vi "Drive.vi"() -> (0 "Front Right":T1={"DeviceStatus"={"status"=FALSE, "code"=0, "source"=""}, "Type"=enum."PWM", "PWM"={"PWM Channel"=enum."PWM 1", "DeadBand"={"Name"="", "maxPositivePwm"=0, "minPositivePwm"=0, "centerPwm"=0, "maxNegativePwm"=0, "minNegativePwm"=0, "angularRange"=0}}, "CAN"={"Device Number"=0, "SetOutput VI Ref"=variant(enum8{"Percent VBus", "Current", "Speed", "Position", "Voltage"} enum."Percent VBus"), "GetOutput VI Ref"=variant(refnum<k1> refnum), "Enable VI Ref"=variant(dbl 12.0), "Disable VI Ref"=variant(enum8{"Percent VBus", "Speed", "Position", "Slave", "Unchanged / Invalid", "Voltage Compensation", "Current", "Motion Profile"} enum."Percent VBus"), "Data"=variant}, "Invert"=FALSE, "DIO PWM"={"PWM \"Enable\" Channel"=enum."Invalid", "DIOChannel"=enum."Invalid", "PWM Rate"=0.0}}, 1 "Front Left":T1={"DeviceStatus"={"status"=FALSE, "code"=0, "source"=""}, "Type"=enum."PWM", "PWM"={"PWM Channel"=enum."PWM 1", "DeadBand"={"Name"="", "maxPositivePwm"=0, "minPositivePwm"=0, "centerPwm"=0, "maxNegativePwm"=0, "minNegativePwm"=0, "angularRange"=0}}, "CAN"={"Device Number"=0, "SetOutput VI Ref"=variant(enum8{"Percent VBus", "Current", "Speed", "Position", "Voltage"} enum."Percent VBus"), "GetOutput VI Ref"=variant(refnum<k1> refnum), "Enable VI Ref"=variant(dbl 12.0), "Disable VI Ref"=variant(enum8{"Percent VBus", "Speed", "Position", "Slave", "Unchanged / Invalid", "Voltage Compensation", "Current", "Motion Profile"} enum."Percent VBus"), "Data"=variant}, "Invert"=FALSE, "DIO PWM"={"PWM \"Enable\" Channel"=enum."Invalid", "DIOChannel"=enum."Invalid", "PWM Rate"=0.0}}, 2 "Rear Right":T1={"DeviceStatus"={"status"=FALSE, "code"=0, "source"=""}, "Type"=enum."PWM", "PWM"={"PWM Channel"=enum."PWM 1", "DeadBand"={"Name"="", "maxPositivePwm"=0, "minPositivePwm"=0, "centerPwm"=0, "maxNegativePwm"=0, "minNegativePwm"=0, "angularRange"=0}}, "CAN"={"Device Number"=0, "SetOutput VI Ref"=variant(enum8{"Percent VBus", "Current", "Speed", "Position", "Voltage"} enum."Percent VBus"), "GetOutput VI Ref"=variant(refnum<k1> refnum), "Enable VI Ref"=variant(dbl 12.0), "Disable VI Ref"=variant(enum8{"Percent VBus", "Speed", "Position", "Slave", "Unchanged / Invalid", "Voltage Compensation", "Current", "Motion Profile"} enum."Percent VBus"), "Data"=variant}, "Invert"=FALSE, "DIO PWM"={"PWM \"Enable\" Channel"=enum."Invalid", "DIOChannel"=enum."Invalid", "PWM Rate"=0.0}}, 3 "Rear Left":T1={"DeviceStatus"={"status"=FALSE, "code"=0, "source"=""}, "Type"=enum."PWM", "PWM"={"PWM Channel"=enum."PWM 1", "DeadBand"={"Name"="", "maxPositivePwm"=0, "minPositivePwm"=0, "centerPwm"=0, "maxNegativePwm"=0, "minNegativePwm"=0, "angularRange"=0}}, "CAN"={"Device Number"=0, "SetOutput VI Ref"=variant(enum8{"Percent VBus", "Current", "Speed", "Position", "Voltage"} enum."Percent VBus"), "GetOutput VI Ref"=variant(refnum<k1> refnum), "Enable VI Ref"=variant(dbl 12.0), "Disable VI Ref"=variant(enum8{"Percent VBus", "Speed", "Position", "Slave", "Unchanged / Invalid", "Voltage Compensation", "Current", "Motion Profile"} enum."Percent VBus"), "Data"=variant}, "Invert"=FALSE, "DIO PWM"={"PWM \"Enable\" Channel"=enum."Invalid", "DIOChannel"=enum."Invalid", "PWM Rate"=0.0}})   [LabVIEW 2019]
uses:
  <vilib>/Rock Robotics/WPI/MotorControl/WPI_MotorControlDeviceRef.ctl
  <vilib>/Rock Robotics/WPI/MotorControl/WPI_MotorControlType.ctl
  <vilib>/Rock Robotics/SystemInterfaces/DIO/FPGA_DIOPWMChannel.ctl
  <vilib>/Rock Robotics/WPI/PWM/WPI_PWMDeadband.ctl
  <vilib>/Rock Robotics/SystemInterfaces/DIO/FPGA_DIOChannel.ctl
  <vilib>/Rock Robotics/WPI/ThirdParty/Phoenix-LabVIEW/Motor Controller/Controls/CTRE_Phoenix_MotorControl_ControlMode.ctl
  <vilib>/Rock Robotics/WPI/ThirdParty/Phoenix-LabVIEW/Motor Controller/Controls/CTRE_Phoenix_MotorControl_FeedbackDevice_TalonFX.ctl
  <vilib>/Rock Robotics/WPI/ThirdParty/Phoenix-LabVIEW/Motor Controller/Controls/CTRE_Phoenix_MotorControl_NeutralMode.ctl
  <vilib>/Rock Robotics/WPI/ThirdParty/Phoenix-LabVIEW/CANCoder/Controls/CTRE_Phoenix_CANcoder_SensorInitializationStrategy.ctl
  <vilib>/Rock Robotics/WPI/ThirdParty/Phoenix-LabVIEW/Motor Controller/Sensor/CTRE_Phoenix_MotorControl_SetIntegratedSensorPosition_TalonFX.vi
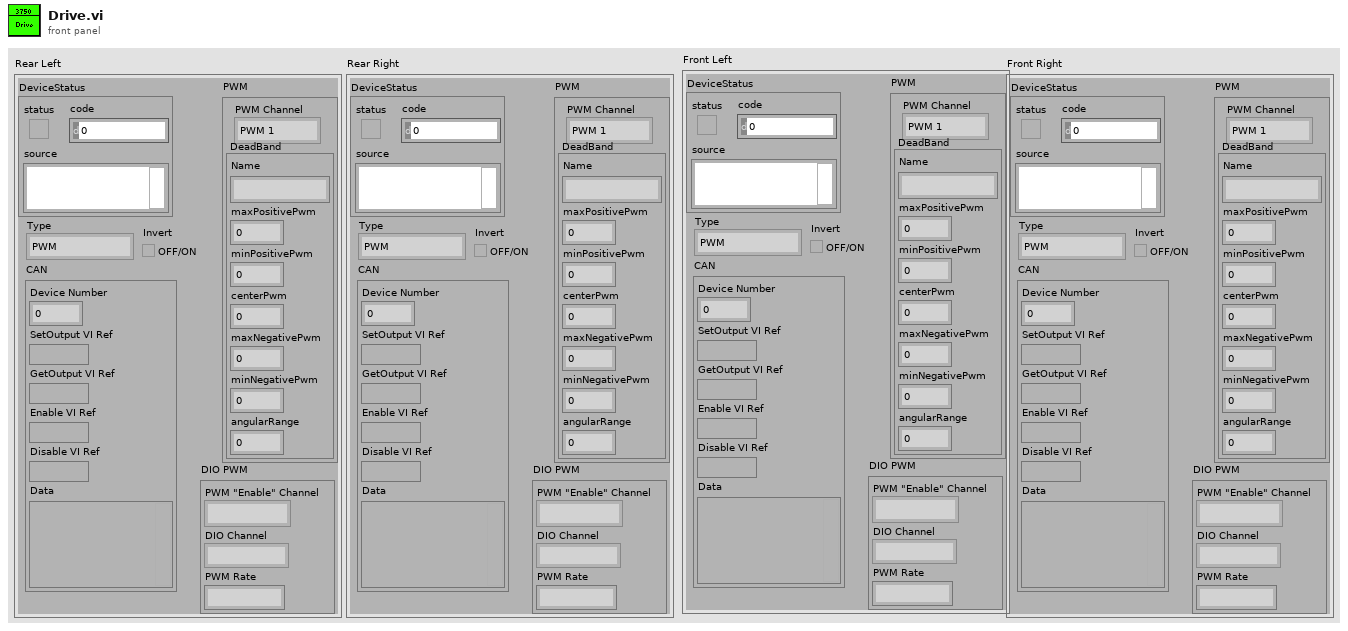
[diagram p1: front panel]
types:
  T1 = typedef "WPI_MotorControlDeviceRef.ctl" = cluster{"DeviceStatus":errorcluster, "Type":T2, "PWM":cluster{"PWM Channel":T3, "DeadBand":T4}, "CAN":cluster{"Device Number":u8, "SetOutput VI Ref":variant, "GetOutput VI Ref":variant, "Enable VI Ref":variant, "Disable VI Ref":variant, "Data":variant}, "Invert":bool, "DIO PWM":cluster{"PWM \"Enable\" Channel":T3, "DIOChannel":T5, "PWM Rate":dbl}}
  T2 = typedef "WPI_MotorControlType.ctl" = enum16{"PWM", "CAN", "DIO PWM"}
  T3 = typedef "FPGA_DIOPWMChannel.ctl" = enum8{"PWM 0", "PWM 1", "PWM 2", "PWM 3", "PWM 4", "PWM 5", "PWM 6", "PWM 7", "PWM 8", "PWM 9", "PWM MXP 0", "PWM MXP 1", "PWM MXP 2", "PWM MXP 3", "PWM MXP 4", "PWM MXP 5", "PWM MXP 6", "PWM MXP 7", "PWM MXP 8", "PWM MXP 9", "Invalid"}
  T4 = typedef "WPI_PWMDeadband.ctl" = cluster{"Name":string, "maxPositivePwm":i32, "minPositivePwm":i32, "centerPwm":i32, "maxNegativePwm":i32, "minNegativePwm":i32, "angularRange":u16}
  T5 = typedef "FPGA_DIOChannel.ctl" = enum8{"DIO 0", "DIO 1", "DIO 2", "DIO 3", "DIO 4", "DIO 5", "DIO 6", "DIO 7", "DIO 8", "DIO 9", "DIO MXP 0", "DIO MXP 1", "DIO MXP 2", "DIO MXP 3", "DIO MXP 4", "DIO MXP 5", "DIO MXP 6", "DIO MXP 7", "DIO MXP 8", "DIO MXP 9", "DIO MXP 10", "DIO MXP 11", "DIO MXP 12", "DIO MXP 13", "DIO MXP 14", "DIO MXP 15", "SPI Port CS1", "SPI Port CS2", "SPI Port CS3", "SPI Port MISO", "SPI Port MOSI", "Invalid"}
  T6 = typedef "CTRE_Phoenix_CANcoder_SensorInitializationStrategy.ctl" = enum16{"Boot To Zero", "Boot To Absolute Position"}
  T7 = typedef "CTRE_Phoenix_MotorControl_NeutralMode.ctl" = enum8{"EEPROMSetting", "Override to Coast", "Override to Brake"}
  T8 = typedef "CTRE_Phoenix_MotorControl_FeedbackDevice_TalonFX.ctl" = i8
  T9 = typedef "CTRE_Phoenix_MotorControl_ControlMode.ctl" = u16
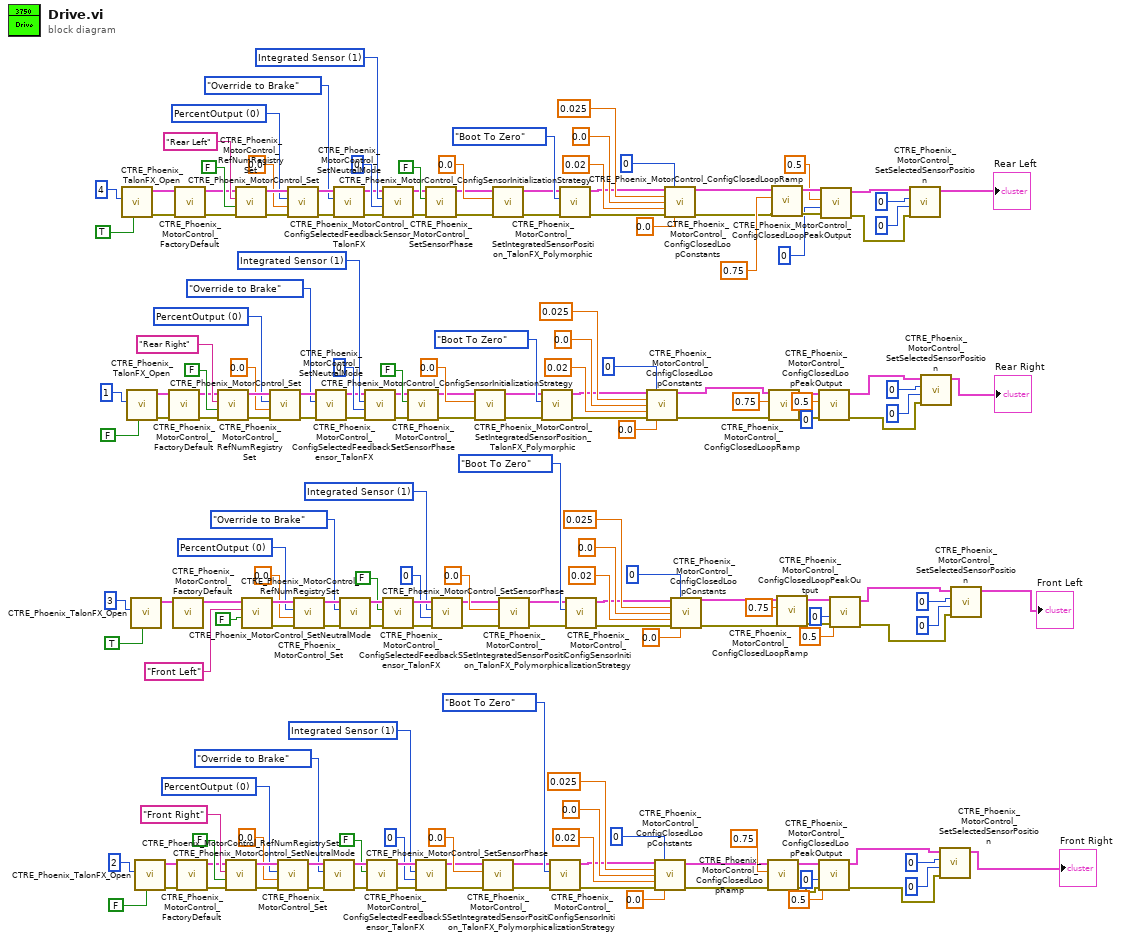
[diagram p0: block diagram]
diagram:
  w134 = T8 1 items=["Integrated Sensor"=1, "Sensor Sum (S0 + S1)"=9, "Sensor Difference (D0 - D1)"=10, "Remote Source 0"=11, "Remote Source 1"=12, "None"=14, "Software Emulated"=15] ("Talon FX Feedback Device")
  w137 = T9 0 items=["PercentOutput"=0, "Position"=1, "Velocity"=2, "Current"=3, "Follower"=5, "MotionProfile"=6, "MotionMagic"=7, "MotionProfileArc"=10, "Disabled"=15] ("Control Mode")
  w150 = T8 1 items=["Integrated Sensor"=1, "Sensor Sum (S0 + S1)"=9, "Sensor Difference (D0 - D1)"=10, "Remote Source 0"=11, "Remote Source 1"=12, "None"=14, "Software Emulated"=15] ("Talon FX Feedback Device")
  w153 = T9 0 items=["PercentOutput"=0, "Position"=1, "Velocity"=2, "Current"=3, "Follower"=5, "MotionProfile"=6, "MotionMagic"=7, "MotionProfileArc"=10, "Disabled"=15] ("Control Mode")
  w166 = T8 1 items=["Integrated Sensor"=1, "Sensor Sum (S0 + S1)"=9, "Sensor Difference (D0 - D1)"=10, "Remote Source 0"=11, "Remote Source 1"=12, "None"=14, "Software Emulated"=15] ("Talon FX Feedback Device")
  w168 = T9 0 items=["PercentOutput"=0, "Position"=1, "Velocity"=2, "Current"=3, "Follower"=5, "MotionProfile"=6, "MotionMagic"=7, "MotionProfileArc"=10, "Disabled"=15] ("Control Mode")
  w177 = T8 1 items=["Integrated Sensor"=1, "Sensor Sum (S0 + S1)"=9, "Sensor Difference (D0 - D1)"=10, "Remote Source 0"=11, "Remote Source 1"=12, "None"=14, "Software Emulated"=15] ("Talon FX Feedback Device")
  w179 = T9 0 items=["PercentOutput"=0, "Position"=1, "Velocity"=2, "Current"=3, "Follower"=5, "MotionProfile"=6, "MotionMagic"=7, "MotionProfileArc"=10, "Disabled"=15] ("Control Mode")
  n1 = call <vilib>:"CTRE_Phoenix_TalonFX_Open.vi"("Invert"=TRUE, "Device Number"=u8 4) -> ("error out"=w74:errorcluster, "CAN Talon SRX Ref"=w76:T1)  [unwired: 8 in]
  n2 = call <vilib>:"CTRE_Phoenix_TalonFX_Open.vi"("Invert"=FALSE, "Device Number"=u8 1) -> ("error out"=w70:errorcluster, "CAN Talon SRX Ref"=w72:T1)  [unwired: 8 in]
  n3 = call <vilib>:"CTRE_Phoenix_TalonFX_Open.vi"("Invert"=TRUE, "Device Number"=u8 3) -> ("CAN Talon SRX Ref"=w68:T1)  [unwired: 8 in, 1 out]
  n4 = call <vilib>:"CTRE_Phoenix_TalonFX_Open.vi"("Invert"=FALSE, "Device Number"=u8 2) -> ("error out"=w64:errorcluster, "CAN Talon SRX Ref"=w66:T1)  [unwired: 8 in]
  n5 = call <vilib>:"CTRE_Phoenix_MotorControl_FactoryDefault.vi"("error in"=w70, "PhoenixMotorControlDevRef"=w72) -> ("error out"=w69:errorcluster, "PhoenixMotorControlDevRef"=w71:T1)  [unwired: 8 in]
  n6 = call <vilib>:"CTRE_Phoenix_MotorControl_FactoryDefault.vi"("PhoenixMotorControlDevRef"=w68) -> ("PhoenixMotorControlDevRef"=w67:T1)  [unwired: 9 in, 1 out]
  n7 = call <vilib>:"CTRE_Phoenix_MotorControl_FactoryDefault.vi"("error in"=w74, "PhoenixMotorControlDevRef"=w76) -> ("error out"=w73:errorcluster, "PhoenixMotorControlDevRef"=w75:T1)  [unwired: 8 in]
  n8 = call <vilib>:"CTRE_Phoenix_MotorControl_FactoryDefault.vi"("error in"=w64, "PhoenixMotorControlDevRef"=w66) -> ("error out"=w63:errorcluster, "PhoenixMotorControlDevRef"=w65:T1)  [unwired: 8 in]
  n9 = call <vilib>:"CTRE_Phoenix_MotorControl_RefNumRegistrySet.vi"("error in (no error)"=w69, "Test Mode Only"=FALSE, "refnum name"="Rear Right", "PhoenixMotorControlDevRef"=w71) -> ("error out"=w175:errorcluster, "PhoenixMotorControlDevRef"=w174:T1)  [unwired: 6 in]
  n10 = call <vilib>:"CTRE_Phoenix_MotorControl_RefNumRegistrySet.vi"("error in (no error)"=w63, "Test Mode Only"=FALSE, "refnum name"="Front Right", "PhoenixMotorControlDevRef"=w65) -> ("error out"=w148:errorcluster, "PhoenixMotorControlDevRef"=w147:T1)  [unwired: 6 in]
  n11 = call <vilib>:"CTRE_Phoenix_MotorControl_RefNumRegistrySet.vi"("error in (no error)"=w73, "Test Mode Only"=FALSE, "refnum name"="Rear Left", "PhoenixMotorControlDevRef"=w75) -> ("error out"=w186:errorcluster, "PhoenixMotorControlDevRef"=w185:T1)  [unwired: 6 in]
  n12 = call <vilib>:"CTRE_Phoenix_MotorControl_RefNumRegistrySet.vi"("Test Mode Only"=FALSE, "refnum name"="Front Left", "PhoenixMotorControlDevRef"=w67) -> ("error out"=w164:errorcluster, "PhoenixMotorControlDevRef"=w163:T1)  [unwired: 7 in]
  n13 = call <vilib>:"CTRE_Phoenix_MotorControl_Set.vi"("error in (no error)"=w175, "Output"=0.0, "Control Mode"=w168, "PhoenixMotorControlDevRef"=w174) -> ("error out"=w173:errorcluster, "PhoenixMotorControlDevRef"=w172:T1)  [unwired: 6 in]
  n14 = call <vilib>:"CTRE_Phoenix_MotorControl_Set.vi"("error in (no error)"=w148, "Output"=0.0, "Control Mode"=w137, "PhoenixMotorControlDevRef"=w147) -> ("error out"=w146:errorcluster, "PhoenixMotorControlDevRef"=w145:T1)  [unwired: 6 in]
  n15 = call <vilib>:"CTRE_Phoenix_MotorControl_Set.vi"("error in (no error)"=w186, "Output"=0.0, "Control Mode"=w179, "PhoenixMotorControlDevRef"=w185) -> ("error out"=w184:errorcluster, "PhoenixMotorControlDevRef"=w183:T1)  [unwired: 6 in]
  n16 = call <vilib>:"CTRE_Phoenix_MotorControl_Set.vi"("error in (no error)"=w164, "Output"=0.0, "Control Mode"=w153, "PhoenixMotorControlDevRef"=w163) -> ("error out"=w162:errorcluster, "PhoenixMotorControlDevRef"=w161:T1)  [unwired: 6 in]
  n17 = call <vilib>:"CTRE_Phoenix_MotorControl_SetNeutralMode.vi"("error in (no error)"=w173, "Motor Control Neutral Mode"=CTRE_Phoenix_MotorControl_NeutralMode."Override to Brake", "PhoenixMotorControlDevRef"=w172) -> ("error out"=w61:errorcluster, "PhoenixMotorControlDevRef"=w62:T1)  [unwired: 7 in]
  n18 = call <vilib>:"CTRE_Phoenix_MotorControl_SetNeutralMode.vi"("error in (no error)"=w146, "Motor Control Neutral Mode"=CTRE_Phoenix_MotorControl_NeutralMode."Override to Brake", "PhoenixMotorControlDevRef"=w145) -> ("error out"=w144:errorcluster, "PhoenixMotorControlDevRef"=w143:T1)  [unwired: 7 in]
  n19 = call <vilib>:"CTRE_Phoenix_MotorControl_SetNeutralMode.vi"("error in (no error)"=w184, "Motor Control Neutral Mode"=CTRE_Phoenix_MotorControl_NeutralMode."Override to Brake", "PhoenixMotorControlDevRef"=w183) -> ("error out"=w54:errorcluster, "PhoenixMotorControlDevRef"=w55:T1)  [unwired: 7 in]
  n20 = call <vilib>:"CTRE_Phoenix_MotorControl_SetNeutralMode.vi"("error in (no error)"=w162, "Motor Control Neutral Mode"=CTRE_Phoenix_MotorControl_NeutralMode."Override to Brake", "PhoenixMotorControlDevRef"=w161) -> ("error out"=w160:errorcluster, "PhoenixMotorControlDevRef"=w159:T1)  [unwired: 7 in]
  n21 = call <vilib>:"CTRE_Phoenix_MotorControl_ConfigSelectedFeedbackSensor_TalonFX.vi"("error in (no error)"=w61, "pidLoopIdx"=0, "Talon FX Feedback Device"=w166, "PhoenixMotorControlDevRef"=w62) -> ("error out"=w56:errorcluster, "PhoenixMotorControlDevRef"=w57:T1)  [unwired: 6 in]
  n22 = call <vilib>:"CTRE_Phoenix_MotorControl_SetSensorPhase.vi"("error in (no error)"=w144, "PhaseSensor"=FALSE, "PhoenixMotorControlDevRef"=w143) -> ("error out"=w142:errorcluster, "PhoenixMotorControlDevRef"=w141:T1)  [unwired: 7 in]
  n23 = call <vilib>:"CTRE_Phoenix_MotorControl_ConfigSelectedFeedbackSensor_TalonFX.vi"("error in (no error)"=w54, "pidLoopIdx"=0, "Talon FX Feedback Device"=w177, "PhoenixMotorControlDevRef"=w55) -> ("error out"=w51:errorcluster, "PhoenixMotorControlDevRef"=w52:T1)  [unwired: 6 in]
  n24 = call <vilib>:"CTRE_Phoenix_MotorControl_SetSensorPhase.vi"("error in (no error)"=w160, "PhaseSensor"=FALSE, "PhoenixMotorControlDevRef"=w159) -> ("error out"=w158:errorcluster, "PhoenixMotorControlDevRef"=w157:T1)  [unwired: 7 in]
  n25 = call <vilib>:"CTRE_Phoenix_MotorControl_SetSensorPhase.vi"("error in (no error)"=w56, "PhaseSensor"=FALSE, "PhoenixMotorControlDevRef"=w57) -> ("error out"=w58:errorcluster, "PhoenixMotorControlDevRef"=w59:T1)  [unwired: 7 in]
  n26 = call <vilib>:"CTRE_Phoenix_MotorControl_ConfigSelectedFeedbackSensor_TalonFX.vi"("error in (no error)"=w142, "pidLoopIdx"=0, "Talon FX Feedback Device"=w134, "PhoenixMotorControlDevRef"=w141) -> ("error out"=w80:errorcluster, "PhoenixMotorControlDevRef"=w77:T1)  [unwired: 6 in]
  n27 = call <vilib>:"CTRE_Phoenix_MotorControl_SetSensorPhase.vi"("error in (no error)"=w51, "PhaseSensor"=FALSE, "PhoenixMotorControlDevRef"=w52) -> ("error out"=w49:errorcluster, "PhoenixMotorControlDevRef"=w50:T1)  [unwired: 7 in]
  n28 = call <vilib>:"CTRE_Phoenix_MotorControl_ConfigSelectedFeedbackSensor_TalonFX.vi"("error in (no error)"=w158, "pidLoopIdx"=0, "Talon FX Feedback Device"=w150, "PhoenixMotorControlDevRef"=w157) -> ("error out"=w85:errorcluster, "PhoenixMotorControlDevRef"=w82:T1)  [unwired: 6 in]
  n29 = call-poly <vilib>:"CTRE_Phoenix_MotorControl_SetIntegratedSensorPosition_TalonFX_Polymorphic.vi"("error in (no error)"=w58, "New Position"=0.0, "PhoenixMotorControlDevRef"=w59) -> ("error out"=w87:errorcluster, "PhoenixMotorControlDevRef"=w88:T1)  [unwired: 7 in]
  n30 = call-poly <vilib>:"CTRE_Phoenix_MotorControl_SetIntegratedSensorPosition_TalonFX_Polymorphic.vi"("error in (no error)"=w80, "New Position"=0.0, "PhoenixMotorControlDevRef"=w77) -> ("error out"=w79:errorcluster, "PhoenixMotorControlDevRef"=w78:T1)  [unwired: 7 in]
  n31 = call-poly <vilib>:"CTRE_Phoenix_MotorControl_SetIntegratedSensorPosition_TalonFX_Polymorphic.vi"("error in (no error)"=w49, "New Position"=0.0, "PhoenixMotorControlDevRef"=w50) -> ("error out"=w91:errorcluster, "PhoenixMotorControlDevRef"=w90:T1)  [unwired: 7 in]
  n32 = call-poly <vilib>:"CTRE_Phoenix_MotorControl_SetIntegratedSensorPosition_TalonFX_Polymorphic.vi"("error in (no error)"=w85, "New Position"=0.0, "PhoenixMotorControlDevRef"=w82) -> ("error out"=w84:errorcluster, "PhoenixMotorControlDevRef"=w83:T1)  [unwired: 7 in]
  n33 = call <vilib>:"CTRE_Phoenix_MotorControl_ConfigSensorInitializationStrategy.vi"("error in (no error)"=w87, "Sensor Initialization Strategy"=CTRE_Phoenix_CANcoder_SensorInitializationStrategy."Boot To Zero", "PhoenixMotorControlDevRef"=w88) -> ("error out"=w96:errorcluster, "PhoenixMotorControlDevRef"=w97:T1)  [unwired: 7 in]
  n34 = call <vilib>:"CTRE_Phoenix_MotorControl_ConfigSensorInitializationStrategy.vi"("error in (no error)"=w79, "Sensor Initialization Strategy"=CTRE_Phoenix_CANcoder_SensorInitializationStrategy."Boot To Zero", "PhoenixMotorControlDevRef"=w78) -> ("error out"=w103:errorcluster, "PhoenixMotorControlDevRef"=w104:T1)  [unwired: 7 in]
  n35 = call <vilib>:"CTRE_Phoenix_MotorControl_ConfigSensorInitializationStrategy.vi"("error in (no error)"=w91, "Sensor Initialization Strategy"=CTRE_Phoenix_CANcoder_SensorInitializationStrategy."Boot To Zero", "PhoenixMotorControlDevRef"=w90) -> ("error out"=w93:errorcluster, "PhoenixMotorControlDevRef"=w94:T1)  [unwired: 7 in]
  n36 = call <vilib>:"CTRE_Phoenix_MotorControl_ConfigSensorInitializationStrategy.vi"("error in (no error)"=w84, "Sensor Initialization Strategy"=CTRE_Phoenix_CANcoder_SensorInitializationStrategy."Boot To Zero", "PhoenixMotorControlDevRef"=w83) -> ("error out"=w99:errorcluster, "PhoenixMotorControlDevRef"=w100:T1)  [unwired: 7 in]
  n37 = call <vilib>:"CTRE_Phoenix_MotorControl_ConfigClosedLoopConstants.vi"("PhoenixMotorControlDevRef"=w97, "slotIdx"=0, "P"=0.025, "I"=0.0, "D"=0.02, "error in (no error)"=w96, "F"=0.0) -> ("PhoenixMotorControlDevRef"=w24:T1, "error out"=w23:errorcluster)  [unwired: 7 in]
  n38 = call <vilib>:"CTRE_Phoenix_MotorControl_ConfigClosedLoopConstants.vi"("PhoenixMotorControlDevRef"=w104, "slotIdx"=0, "P"=0.025, "I"=0.0, "D"=0.02, "error in (no error)"=w103, "F"=0.0) -> ("PhoenixMotorControlDevRef"=w12:T1, "error out"=w11:errorcluster)  [unwired: 7 in]
  n39 = call <vilib>:"CTRE_Phoenix_MotorControl_ConfigClosedLoopConstants.vi"("PhoenixMotorControlDevRef"=w94, "slotIdx"=0, "P"=0.025, "I"=0.0, "D"=0.02, "error in (no error)"=w93, "F"=0.0) -> ("PhoenixMotorControlDevRef"=w28:T1, "error out"=w27:errorcluster)  [unwired: 7 in]
  n40 = call <vilib>:"CTRE_Phoenix_MotorControl_ConfigClosedLoopConstants.vi"("PhoenixMotorControlDevRef"=w100, "slotIdx"=0, "P"=0.025, "I"=0.0, "D"=0.02, "error in (no error)"=w99, "F"=0.0) -> ("PhoenixMotorControlDevRef"=w10:T1, "error out"=w9:errorcluster)  [unwired: 7 in]
  n41 = call <vilib>:"CTRE_Phoenix_MotorControl_ConfigClosedLoopRamp.vi"("error in (no error)"=w11, "secondsFromNeutralToFull"=0.75, "PhoenixMotorControlDevRef"=w12) -> ("error out"=w31:errorcluster, "PhoenixMotorControlDevRef"=w32:T1)  [unwired: 7 in]
  n42 = call <vilib>:"CTRE_Phoenix_MotorControl_ConfigClosedLoopRamp.vi"("error in (no error)"=w23, "secondsFromNeutralToFull"=0.75, "PhoenixMotorControlDevRef"=w24) -> ("error out"=w39:errorcluster, "PhoenixMotorControlDevRef"=w40:T1)  [unwired: 7 in]
  n43 = call <vilib>:"CTRE_Phoenix_MotorControl_ConfigClosedLoopRamp.vi"("error in (no error)"=w27, "secondsFromNeutralToFull"=0.75, "PhoenixMotorControlDevRef"=w28) -> ("error out"=w43:errorcluster, "PhoenixMotorControlDevRef"=w44:T1)  [unwired: 7 in]
  n44 = call <vilib>:"CTRE_Phoenix_MotorControl_ConfigClosedLoopRamp.vi"("error in (no error)"=w9, "secondsFromNeutralToFull"=0.75, "PhoenixMotorControlDevRef"=w10) -> ("error out"=w36:errorcluster, "PhoenixMotorControlDevRef"=w37:T1)  [unwired: 7 in]
  n45 = call <vilib>:"CTRE_Phoenix_MotorControl_ConfigClosedLoopPeakOutput.vi"("error in (no error)"=w39, "slotIdx"=0, "peakOutput"=0.5, "PhoenixMotorControlDevRef"=w40) -> ("error out"=w5:errorcluster, "PhoenixMotorControlDevRef"=w4:T1)  [unwired: 6 in]
  n46 = call <vilib>:"CTRE_Phoenix_MotorControl_ConfigClosedLoopPeakOutput.vi"("error in (no error)"=w31, "slotIdx"=0, "peakOutput"=0.5, "PhoenixMotorControlDevRef"=w32) -> ("error out"=w6:errorcluster, "PhoenixMotorControlDevRef"=w14:T1)  [unwired: 6 in]
  n47 = call <vilib>:"CTRE_Phoenix_MotorControl_ConfigClosedLoopPeakOutput.vi"("error in (no error)"=w43, "slotIdx"=0, "peakOutput"=0.5, "PhoenixMotorControlDevRef"=w44) -> ("error out"=w3:errorcluster, "PhoenixMotorControlDevRef"=w22:T1)  [unwired: 6 in]
  n48 = call <vilib>:"CTRE_Phoenix_MotorControl_ConfigClosedLoopPeakOutput.vi"("error in (no error)"=w36, "slotIdx"=0, "peakOutput"=0.5, "PhoenixMotorControlDevRef"=w37) -> ("error out"=w7:errorcluster, "PhoenixMotorControlDevRef"=w8:T1)  [unwired: 6 in]
  n49 = call <vilib>:"CTRE_Phoenix_MotorControl_SetSelectedSensorPosition.vi"("error in (no error)"=w3, "pidLoopIdx"=u32 0, "New Sensor Position"=0, "PhoenixMotorControlDevRef"=w22) -> ("PhoenixMotorControlDevRef"=→"Rear Left":T1)  [unwired: 6 in, 1 out]
  n50 = call <vilib>:"CTRE_Phoenix_MotorControl_SetSelectedSensorPosition.vi"("error in (no error)"=w5, "pidLoopIdx"=u32 0, "New Sensor Position"=0, "PhoenixMotorControlDevRef"=w4) -> ("PhoenixMotorControlDevRef"=→"Rear Right":T1)  [unwired: 6 in, 1 out]
  n51 = call <vilib>:"CTRE_Phoenix_MotorControl_SetSelectedSensorPosition.vi"("error in (no error)"=w6, "pidLoopIdx"=u32 0, "New Sensor Position"=0, "PhoenixMotorControlDevRef"=w14) -> ("PhoenixMotorControlDevRef"=→"Front Right":T1)  [unwired: 6 in, 1 out]
  n52 = call <vilib>:"CTRE_Phoenix_MotorControl_SetSelectedSensorPosition.vi"("error in (no error)"=w7, "pidLoopIdx"=u32 0, "New Sensor Position"=0, "PhoenixMotorControlDevRef"=w8) -> ("PhoenixMotorControlDevRef"=→"Front Left":T1)  [unwired: 6 in, 1 out]
